vi "Clear Graph.vi"(11 "Heart Rate Params":T1) -> ()   [LabVIEW 2017]
uses:
  Custom Controls/Heart Rate Parameters.ctl
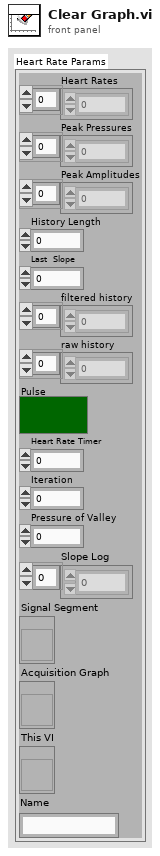
[diagram p1: front panel]
types:
  T1 = typedef "Heart Rate Parameters.ctl" = cluster{"Heart Rates":dbl[], "Peak Pressures":dbl[], "Peak Amplitudes":dbl[], "History Length":i32, "Last  Slope":dbl, "filtered history":dbl[], "raw history":dbl[], "Pulse":bool, "Heart Rate Timer":i32, "Iteration":u32, "Pressure of Valley":dbl, "Slope Log":dbl[], "Signal Segment":refnum<vi>, "Acquisition Graph":refnum<vi>, "This VI":refnum<vi>, "Name":string}
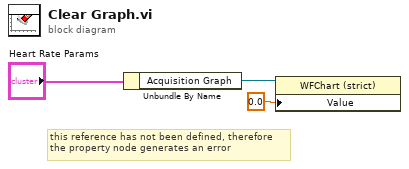
[diagram p0: block diagram]
diagram:
  # "this reference has not been defined, therefore\nthe property node generates an error"
  n1 = Unbundle By Name("Heart Rate Params") -> ("Acquisition Graph"=w2:refnum<vi>)
  n2 = property class="WFChart (strict)"(reference=w2, "Value"=0.0) -> ()  [unwired: 1 in, 2 out]
